vi "MAIN(Autonomous).vi"() -> ()   [LabVIEW 2011]
panel:
  out "Close to Waypoint?":bool
  out "stop 2":bool
  out "New Commands?":bool
  out "Motor Commands":T1(array[cluster])
  in  "stop":bool
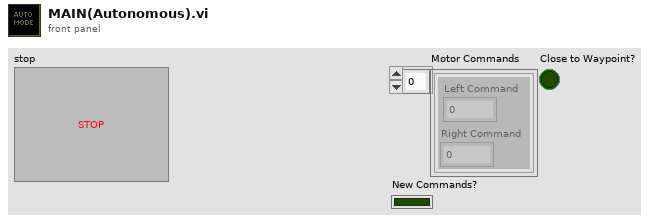
[diagram p1: front panel]
types:
  T1 = cluster{"Left Command":dbl, "Right Command":dbl}[]
  T2 = typedef "IMAQ Image.ctl" = refnum<image>
  T3 = cluster{"Compass Out":refnum<visa-resource-name>, "LIDAR Out":refnum<visa-resource-name>, "GPS Out":refnum<visa-resource-name>, "IMAQ Session Out":refnum<k11>, "Image Out":T2}
  T4 = cluster{"LIDAR Data":cluster{"Magnitude":dbl[], "Direction":dbl[]}, "Line Cam Obstacles":cluster{dbl[], dbl[], i32}}
  T5 = cluster{"compassHeading":dbl, "Robot Position":cluster{"Longitude":dbl, "Latitude":dbl}}
  T6 = cluster{"Compass Out":refnum<visa-resource-name>, "LIDAR Out":refnum<visa-resource-name>, "GPS out":refnum<visa-resource-name>, "IMAQ Session Out":refnum<k11>, "Image (out)":T2}
  T7 = cluster{"x coordinates":i32[], "y coordinates":i32[]}
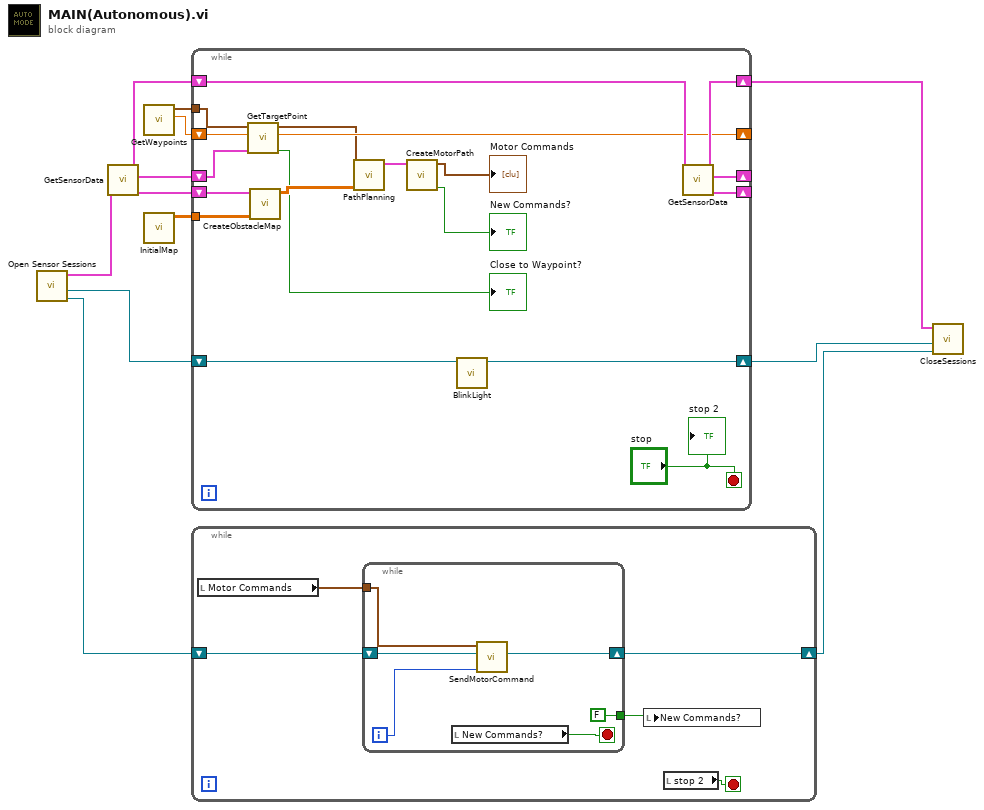
[diagram p0: block diagram]
diagram:
  n1 = call "Open Sensor Sessions.vi"() -> ("Motor out"=w4:refnum<visa-resource-name>, "Relay out"=w12:refnum<visa-resource-name>, "Sensor Sessions"=w10:T3)  [unwired: 9 in]
  n2 = call "GetSensorData.vi"("Sensor Sessions"=w10) -> ("Obstacles"=w8:T4, "Pose"=w9:T5, "Sessions Out"=w11:T6)  [unwired: 8 in]
  n3 = call "GetWaypoints.vi"() -> ("Waypoint Index"=w6:dbl, "Waypoints"=w7:cluster{"Longitude":dbl, "Latitude":dbl}[])  [unwired: 10 in]
  n4 = call "InitialMap.vi"() -> ("Map"=w5:dbl[][])  [unwired: 11 in]
  n5 = while {
    shift-right: [w30] -> w1
    shift-left: w11 -> [w29]
    shift-right: [w25] -> _
    shift-left: w9 -> [w28]
    shift-right: [w24] -> _
    shift-left: w8 -> [w22]
    tunnel: w7 -> [w27]
    shift-right: [w23] -> _
    shift-left: w6 -> [w26]
    tunnel: w5 -> [w18]
    shift-right: [w14] -> w2
    shift-left: w12 -> [w15]
    stop <- "stop" stop-if-true
    n6 = call "GetTargetPoint.vi"("Pose"=w28, "Waypoint Index"=w26, "Waypoints"=w27) -> ("Close to Waypoint?"=→"Close to Waypoint?":bool, "Waypoint Index Out"=w23:dbl, "Target Point"=w21:cluster{"Target X":dbl, "Target  Y":dbl})  [unwired: 6 in]
    n7 = call "CreateObstacleMap.vi"("Base Map"=w18, "Obstacles"=w22) -> ("Obstacle Map"=w20:dbl[][])  [unwired: 9 in]
    n8 = call "PathPlanning.vi"("Obstacle Map"=w20, "Target Point"=w21) -> ("Planned Path"=w19:T7)  [unwired: 9 in]
    n9 = call "CreateMotorPath.vi"("Planned Path"=w19) -> ("New Commands?"=→"New Commands?":bool, "Motor Commands"=→"Motor Commands":T1)  [unwired: 9 in]
    n10 = call "BlinkLight.vi"("Relay In"=w15) -> ("Relay Out"=w14:refnum<visa-resource-name>)  [unwired: 10 in]
    n11 = call "GetSensorData.vi"("Sensor Sessions"=w29) -> ("Obstacles"=w24:T4, "Pose"=w25:T5, "Sessions Out"=w30:T6)  [unwired: 8 in]
    "stop 2" <- "stop"
  }
  n12 = while {
    shift-right: [w32] -> w3
    shift-left: w4 -> [w33]
    stop <- w36 stop-if-true
    n13 = local read "Motor Commands"() -> (w34:T1)
    n14 = while {
      tunnel: [FALSE] -> w35
      tunnel: w34 -> [w40]
      shift-right: [w38] -> w32
      shift-left: w33 -> [w39]
      i -> [w37]
      stop <- w42 stop-if-true
      n15 = local read "New Commands?"() -> (w42:bool)
      n16 = call "SendMotorCommand.vi"("Command Index"=w37, "Motor In"=w39, "Motor Commands"=w40) -> ("Motor Out"=w38:refnum<visa-resource-name>)  [unwired: 8 in]
    }
    n17 = local write "New Commands?"(w35) -> ()
    n18 = local read "stop 2"() -> (w36:bool)
  }
  n19 = call "CloseSessions.vi"("Motor IN"=w3, "Relay In"=w2, "Sessions In"=w1) -> ()  [unwired: 9 in]
